vi "Actor Core.vi"(8 "error in":errorcluster, 11 "Nested in":refnum<class "Database UI.lvclass">) -> (0 "error out":errorcluster, 3 "Actor out":refnum<class "Actor.lvclass">)   [LabVIEW 2023, in "Database UI.lvlib" / "Database UI.lvclass"]
doc: "(<B>Filename</B>: Actor Framework.lvlib:Actor.lvclass:Actor Core.vi)\n\nReceives messages to the actor, reacts to them, and initiates any error handling that may shut the actor down.\n\nDescendant classes may override this VI to append parallel tasks for the actor to complete while it handles messages. Overrides use the Call Parent Method node."
uses:
  Database UI.lvclass
  <vilib>/ActorFramework/Actor/Actor.lvclass
  <vilib>/ActorFramework/Actor/Actor.lvclass/Actor.ctl
  Database UI.lvclass/Database UI.ctl
  Database UI Messages/Read Database Msg/Read Database Msg.lvclass/Read Database Msg.ctl
  <vilib>/ActorFramework/Message Enqueuer/Message Enqueuer.lvclass/Message Enqueuer.ctl
  Database UI Messages/Read Instr CFGs Msg/Read Instr CFGs Msg.lvclass/Read Instr CFGs Msg.ctl
  Configurator/IConfiguration UI Actor/IConfiguration UI Actor Messages/Add Instr CFG Msg/Add Instr CFG Msg.lvclass/Add Instr CFG Msg.ctl
  Configurator/IConfiguration UI Actor/IConfiguration UI Actor Messages/Set Virt Instr CFG Msg/Set Virt Instr CFG Msg.lvclass/Set Virt Instr CFG Msg.ctl
  Configurator/IConfiguration UI Actor/IConfiguration UI Actor Messages/Set Series CFG Msg/Set Series CFG Msg.lvclass/Set Series CFG Msg.ctl
  <vilib>/ActorFramework/Message Enqueuer/Enqueue.vi
  Database UI Messages/Read Database Msg/Read Database Msg.lvclass
  Database UI Messages/Read Instr CFGs Msg/Read Instr CFGs Msg.lvclass
  Configurator/IConfiguration UI Actor/IConfiguration UI Actor Messages/Add Instr CFG Msg/Add Instr CFG Msg.lvclass
  Configurator/IConfiguration UI Actor/IConfiguration UI Actor Messages/Set Virt Instr CFG Msg/Set Virt Instr CFG Msg.lvclass
  Configurator/IConfiguration UI Actor/IConfiguration UI Actor Messages/Set Series CFG Msg/Set Series CFG Msg.lvclass
  <vilib>/Utility/LVClass/Get LV Class Name.vi
  <resource>/AFDebug/Generate Trace for Message.vi
  <vilib>/ActorFramework/Message Priority Queue/Priority Enqueue.vi
  <vilib>/MGI/Panel Manager/Panel Actor/Panel Actor/Panel Actor.lvclass
  C:/Program Files/National Instruments/LabVIEW 2023/vi.lib/MGI/Panel Manager/Panel Actor/Panel Actor/Panel Actor.lvclass
  C:/Program Files/National Instruments/LabVIEW 2023/vi.lib/ActorFramework/Actor/Actor.lvclass
  D:/git/HAL/Database/Database UI/Database UI.lvclass
  D:/git/HAL/Database/IDatabase UI/IDatabase UI/IDatabase UI.lvclass
panel:
  in  "Load":bool
  in  "Series CFGs":string[][](table)
  in  "Series Instr CFGs":string[][](table)
  in  "DB File Path":path=path "D:/git/HAL/Database/configs.db"
  in  "Open Button":bool
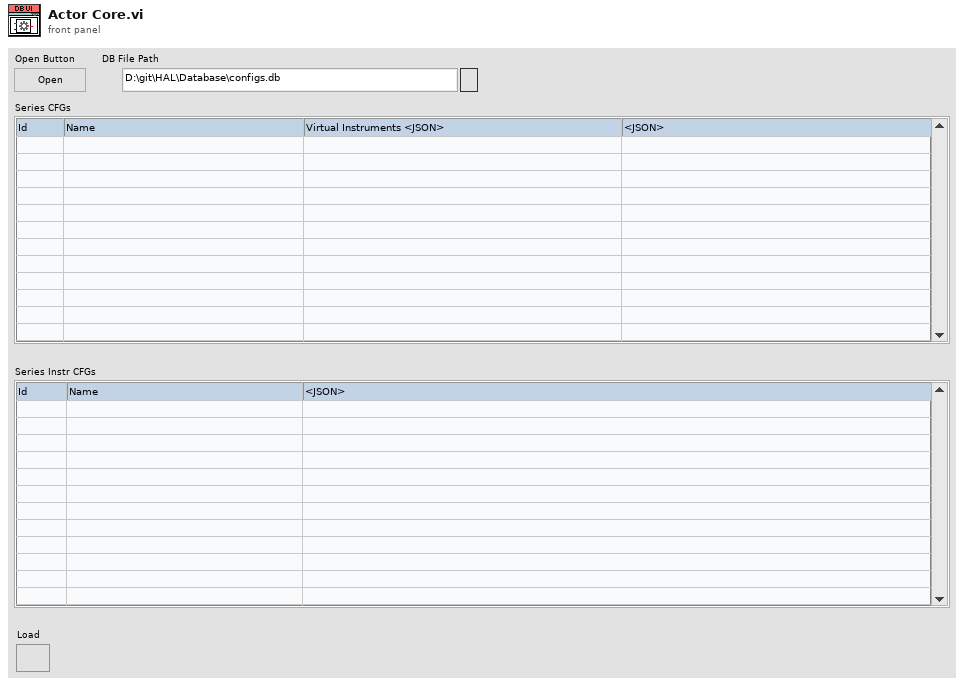
[diagram p1: front panel]
types:
  T1 = cluster{"Series":string, "Virt Instrs":string, "Instrs":string[]}
  T2 = cluster{"Pnl Actor":refnum<event-registration>, "Event Registration Refnum":refnum<event-registration>}
  T3 = typedef "LVPoint32TypeDef.ctl" = cluster{"Horizontal":i32, "Vertical":i32}
  T4 = typedef "LVRowAndColumnTypeDef.ctl" = cluster{"Row":i32, "Column":i32}
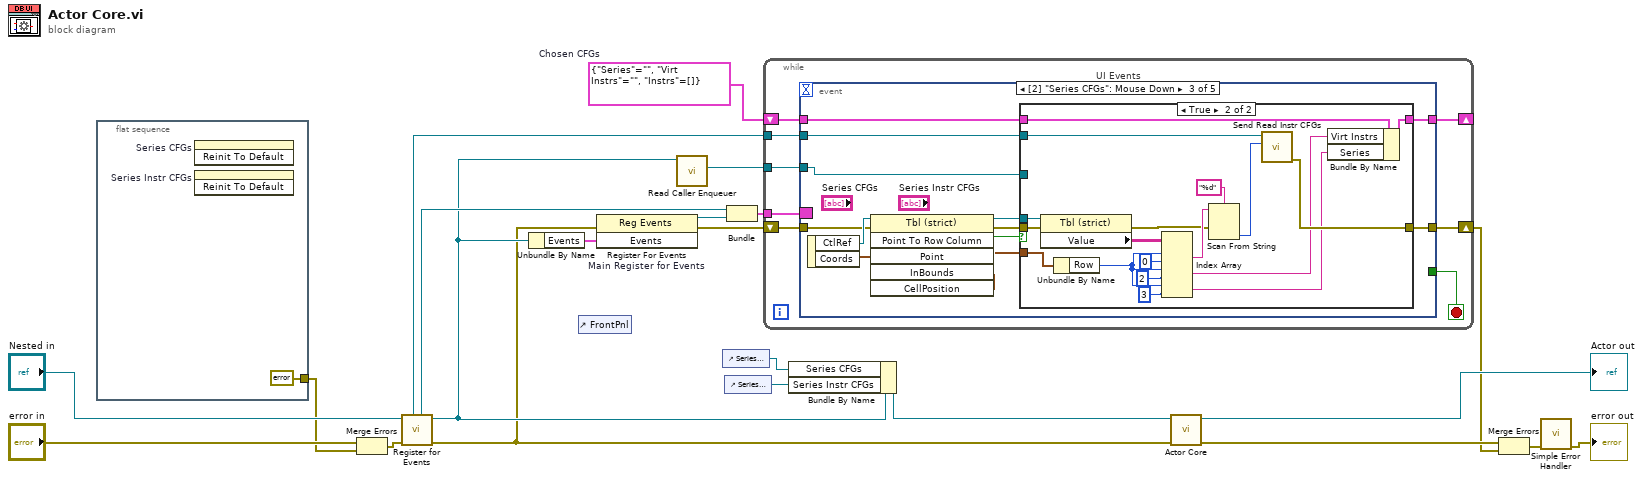
[diagram p0: block diagram]
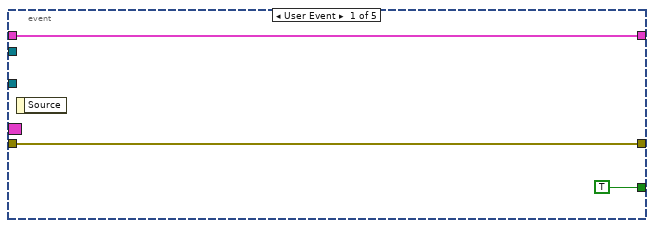
[diagram p2: hidden frame]
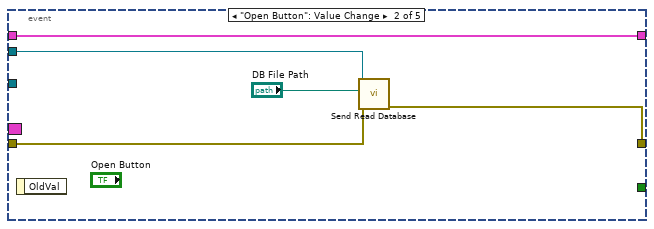
[diagram p3: hidden frame]
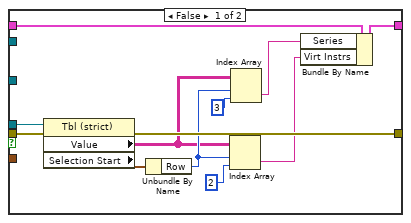
[diagram p4: hidden frame]
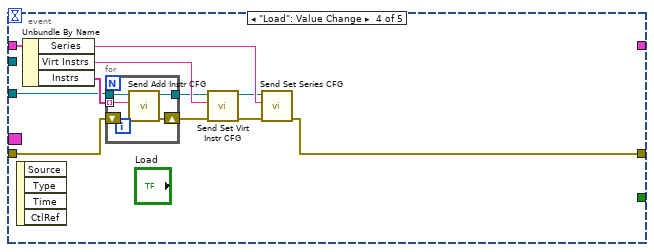
[diagram p5: hidden frame]
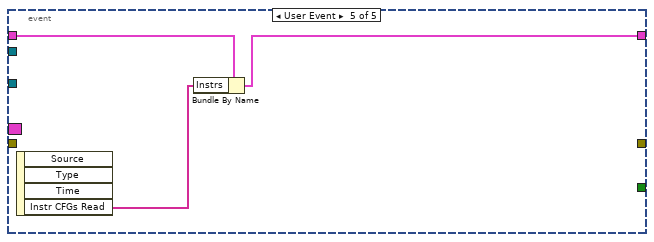
[diagram p6: hidden frame]
diagram:
  w10 = T1 {"Series"="", "Virt Instrs"="", "Instrs"=[]}  # Chosen CFGs
  n1 = flat-sequence {
    tunnel: [errorcluster {"status"=FALSE, "code"=0, "source"=""} ("error in (no error)")] -> w1
    frame #0 {
      n2 = invoke on="Series CFGs" class="Tbl (strict)" method="Reinit To Default"() -> ()  [unwired: 3 in, 3 out]
      n3 = invoke on="Series Instr CFGs" class="Tbl (strict)" method="Reinit To Default"() -> ()  [unwired: 3 in, 3 out]
    }
  }
  n4 = Merge Errors("error in", w1) -> (w2:errorcluster)
  n5 = call <vilib>:"Register for Events.vi"("Error In"=w2, "Panel Actor in"="Nested in") -> ("Error Out"=w8:errorcluster, "Panel Actor out"=w12:refnum<class "Database UI.lvclass">, "Pnl Actor"=w15:refnum<event-registration>, "Self Enqueuer"=w17:refnum<class "Message Enqueuer.lvclass">)  [unwired: 6 in]
  n6 = Unbundle By Name(w12) -> ("Events"=w19:cluster{"Instr CFGs Read":refnum<user-event>})
  n7 = control-ref of="FrontPnl"() -> ()  [unwired: 1 out]
  n8 = register-events "Main Register for Events"(error in=w8, w19) -> (reference out=w20:refnum<event-registration>, error out=w9:errorcluster)  [unwired: 1 in]
  n9 = call <vilib>:"Read Caller Enqueuer.vi"("Actor"=w12) -> ("Caller Enqueuer"=w11:refnum<class "Message Enqueuer.lvclass">)  [unwired: 10 in]
  n10 = control-ref of="Series CFGs"() -> (w7:refnum<vi>)
  n11 = control-ref of="Series Instr CFGs"() -> (w13:refnum<vi>)
  n12 = Bundle("Pnl Actor"=w15, "Event Registration Refnum"=w20) -> (w16:T2)  [unwired: 1 in]
  n13 = while {
    tunnel: w16 -> [w31]
    tunnel: w17 -> [w29]
    tunnel: w11 -> [w28]
    shift-right: [w26] -> _
    shift-left: w10 -> [w27]
    shift-right: [w24] -> w5
    shift-left: w9 -> [w25]
    stop <- w30 stop-if-true
    n14 = event "UI Events" shown="[2] \"Series CFGs\": Mouse Down" {
      selector: w31 -> [_ _ _ _ _]
      dyn-events: _ -> [_ _ _ _ _]
      timeout: _ -> [_ _ _ _ _]
      tunnel: [TRUE _ _ _ _] -> w30
      tunnel: w29 -> [_ w39 w49 _ _]
      tunnel: w28 -> [_ _ w40 w89 _]
      tunnel: w27 -> [w33 w35 w46 w92 w100]
      tunnel: [w33 w35 w45 _ w98] -> w26
      tunnel: w25 -> [w32 w37 w43 w83 _]
      tunnel: [w32 w36 w41 w82 _] -> w24
      event User Event {
        n15 = event-data() -> ()  [unwired: 1 in, 1 out]
      }
      event "Open Button": Value Change {
        n16 = event-data() -> ()  [unwired: 1 in, 1 out]
        n17 = call "Send Read Database.vi"("error in (no error)"=w37, "DB File Path"="DB File Path", "Message Enqueuer"=w39) -> ("error out"=w36:errorcluster)  [unwired: 7 in, 1 out]
      }
      event "Series CFGs": Mouse Down {
        n18 = event-data() -> ("CtlRef"=w48:refnum<vi>, "Coords"=w47:T3)  [unwired: 1 in]
        n19 = invoke class="Tbl (strict)" method="Point To Row Column"(reference=w48, error in=w43, "Point"=w47) -> (reference out=w44:refnum<vi>, error out=w42:errorcluster, "InBounds"=w51:bool, "CellPosition"=w50:T4)  [unwired: 3 in, 2 out]
        n20 = case shown="True" w51 {
          tunnel: w50 -> [_ w81]
          tunnel: w49 -> [_ w74]
          tunnel: w46 -> [w63 w79]
          tunnel: [w59 w78] -> w45
          tunnel: w44 -> [w62 w77]
          tunnel: w42 -> [w58 w76]
          tunnel: [w57 w70] -> w41
          tunnel: w40 -> [_ _]
          frame False {
            n21 = property class="Tbl (strict)"(reference=w62, error in=w58) -> (error out=w57:errorcluster, "Value"=w55:string[][], "Selection Start"=w61:T4)  [unwired: 1 out]
            n22 = Unbundle By Name(w61) -> ("Row"=w56:i32)
            n23 = Index Array(array=w55, index (row)=w56, index (col)=2) -> (element=w53:string)
            n24 = Index Array(array=w55, index (row)=w56, index (col)=3) -> (element=w52:string)
            n25 = Bundle By Name(cluster=w63, "Series"=w52, "Virt Instrs"=w53) -> (w59:T1)
          }
          frame True {
            n26 = property class="Tbl (strict)"(reference=w77, error in=w76) -> (error out=w68:errorcluster, "Value"=w75:string[][])  [unwired: 1 out]
            n27 = Unbundle By Name(w81) -> ("Row"=w73:i32)
            n28 = Index Array(array=w75, index (row) #1=w73, index (col) #1=0 ("index (col)"), index (row) #2=w73, index (col) #2=2 ("index (col)"), index (row) #3=w73, index (col) #3=3 ("index (col)")) -> (element #1=w69:string, element #2=w64:string, element #3=w65:string)
            n29 = Scan From String(format string="%d", input string=w69, error in=w68) -> (output 1=w67:u32)  [unwired: 2 in, 3 out]
            n30 = call "Send Read Instr CFGs.vi"("Series Id"=w67, "Message Enqueuer"=w74) -> ("error out"=w70:errorcluster)  [unwired: 8 in, 1 out]
            n31 = Bundle By Name(cluster=w79, "Virt Instrs"=w64, "Series"=w65) -> (w78:T1)
          }
        }
      }
      event "Load": Value Change {
        n32 = event-data() -> ()  [unwired: 1 in, 4 out]
        n33 = Unbundle By Name(w92) -> ("Series"=w87:string, "Virt Instrs"=w91:string, "Instrs"=w90:string[])
        n34 = for {
          tunnel: w90 -> [w97] mode=indexing
          tunnel: w89 -> [w96]
          tunnel: [w95] -> w88
          shift-right: [w94] -> w85
          shift-left: w83 -> [w93]
          n35 = call "Send Add Instr CFG.vi"("error in (no error)"=w93, "Instr Configuration"=w97, "Message Enqueuer"=w96) -> ("error out"=w94:errorcluster, "Message Enqueuer out"=w95:refnum<class "Message Enqueuer.lvclass">)  [unwired: 7 in]
        }
        n36 = call "Send Set Virt Instr CFG.vi"("error in (no error)"=w85, "Virt Instr CFG"=w91, "Message Enqueuer"=w88) -> ("error out"=w84:errorcluster, "Message Enqueuer out"=w86:refnum<class "Message Enqueuer.lvclass">)  [unwired: 7 in]
        n37 = call "Send Set Series CFG.vi"("error in (no error)"=w84, "Series CFG"=w87, "Message Enqueuer"=w86) -> ("error out"=w82:errorcluster)  [unwired: 7 in, 1 out]
      }
      event User Event {
        n38 = event-data() -> ("Instr CFGs Read"=w99:string[])  [unwired: 1 in, 3 out]
        n39 = Bundle By Name(cluster=w100, "Instrs"=w99) -> (w98:T1)
      }
    }
  }
  n40 = Bundle By Name(cluster=w12, "Series CFGs"=w7, "Series Instr CFGs"=w13) -> (w14:refnum<class "Database UI.lvclass">)
  n41 = call-parent "Actor Core.vi"("error in"=w8, "Panel Actor in"=w14) -> ("error out"=w22:errorcluster, "Actor out"=→"Actor out":refnum<class "Actor.lvclass">)  [unwired: 8 in]
  n42 = Merge Errors(w22, w5) -> (w6:errorcluster)
  n43 = call <vilib>:"Simple Error Handler.vi"("error in (no error)"=w6) -> ("error out"=→"error out":errorcluster)  [unwired: 4 in, 4 out]
